vi "Detail Result List BG Color.vi"(10 "all rows":string[][](array[string]), 11 "reference":refnum<vi>) -> ()   [LabVIEW 2019, in "DataBase.lvlib" / "DataBase.lvclass"]
uses:
  DataBase.lvclass
  <vilib>/Utility/miscctls.llb/LVRowAndColumnTypeDef.ctl
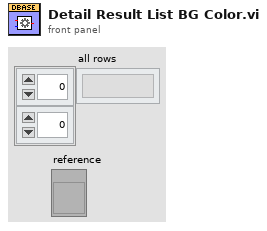
[diagram p1: front panel]
types:
  T1 = typedef "LVRowAndColumnTypeDef.ctl" = cluster{"Row":i32, "Column":i32}
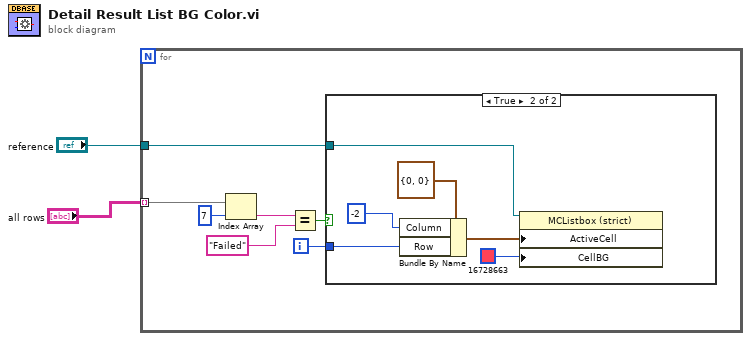
[diagram p0: block diagram]
diagram:
  n1 = for {
    tunnel: "all rows" -> [w5] mode=indexing
    tunnel: "reference" -> [w3]
    i -> [w4]
    n2 = Index Array(array=w5, index=7) -> (element=w7:string)
    n3 = Equal?(x=w7, y="Failed") -> (x = y?=w6:bool)
    n4 = case shown="True" w6 {
      tunnel: w4 -> [_ w11]
      tunnel: w3 -> [_ w10]
      frame False {
      }
      frame True {
        n5 = Bundle By Name(cluster=T1 {"Row"=0, "Column"=0} ("Active Cell:Active Cell"), "Column"=-2, "Row"=w11) -> (w15:T1)
        n6 = property class="MCListbox (strict)"(reference=w10, "ActiveCell"=w15, "CellBG"=u32 16728663 ("Text.Text Colors:Text Color")) -> ()  [unwired: 1 in, 2 out]
      }
    }
  }
